vi "String array to csv.vi"(11 "String Array In":string[](array[string])) -> (3 "CSV String Out":string)   [LabVIEW 2024]
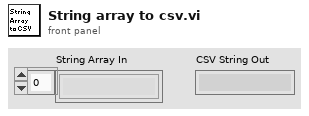
[diagram p1: front panel]
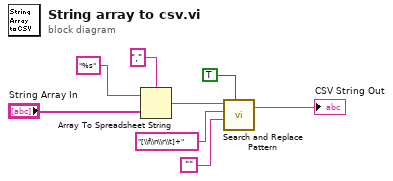
[diagram p0: block diagram]
diagram:
  n1 = Array To Spreadsheet String(delimiter (Tab)=",", array="String Array In", 3:"%s") -> (spreadsheet string=w5:string)
  n2 = call <vilib>:"Search and Replace Pattern.vi"("string"=w5, "regular expression (\"\")"="[\\f\\n\\r\\t]+", "replace string (\"\")"="", "replace all? (F)"=TRUE) -> ("result string"=→"CSV String Out":string)  [unwired: 1 in, 1 out]
